vi "Fibonacci_Sequence_Template.vi"(4 "Sequence Size":i32) -> (1 "Fibonacci Sequence":i32[](array[numeric]))   [LabVIEW 2013]
panel:
  # "Fibonacci Sequence\n\nCreate a VI that takes one numeric input which specifies the number of Fibonacci numbers to\n generate returns an array containing the specified number of numbers of Fibonacci sequence."
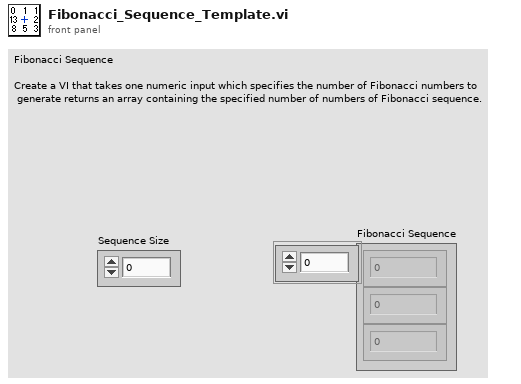
[diagram p1: front panel]
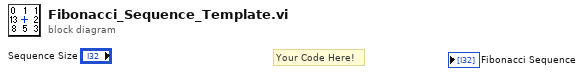
[diagram p0: block diagram]
diagram:
  # "Your Code Here!"
